vi "Motor Controller Config PID.vi"(0 "COM port":refnum<visa-resource-name>, 5 "RS-485 addr.":u8, 7 "Command":string(combo)="Q", 9 "PID params":T1={"N bits"=13, "dt (s)"=0.002, "Kp (/rpm)"=0.002, "Ti (s)"=0.01, "Td (s)"=0.0} {"N bits" min=8 max=16 step=1; "Td (s)" format="%#_6f"; "Ti (s)" format="%#_6f"; "Kp (/rpm)" format="%#_6f"; "dt (s)" format="%#_6f"}, 11 "Set as power-on default":bool, 12 "Close port after action":bool) -> (4 "COM port out":refnum<visa-resource-name>, 15 "Error out":errorcluster)   [LabVIEW 2020]
uses:
  ctls/CTRL_PID_params.ctl
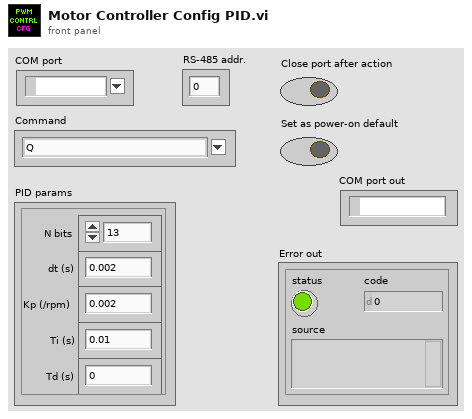
[diagram p1: front panel]
types:
  T1 = typedef "CTRL_PID_params.ctl" = cluster{"N bits":u8, "dt (s)":sgl, "Kp (/rpm)":sgl, "Ti (s)":sgl, "Td (s)":sgl}
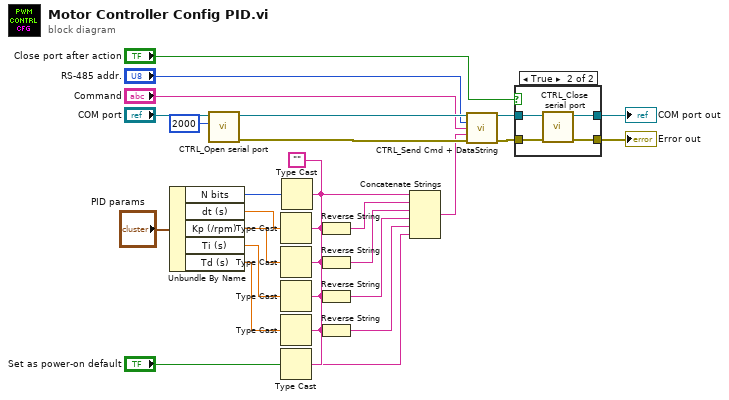
[diagram p0: block diagram]
diagram:
  w5 = ""
  n1 = Unbundle By Name("PID params") -> ("N bits"=w8:u8, "dt (s)"=w14:sgl, "Kp (/rpm)"=w13:sgl, "Ti (s)"=w12:sgl, "Td (s)"=w11:sgl)
  n2 = call "CTRL_Open serial port.vi"("timeout (ms)"=u32 2000, "VISA resource name"="COM port") -> ("Error out"=w27:errorcluster, "VISA resource name out"=w28:refnum<visa-resource-name>)  [unwired: 8 in]
  n3 = Type Cast(type=w5, x=w14) -> (*(type *) &x=w22:string)
  n4 = Type Cast(type=w5, x=w13) -> (*(type *) &x=w21:string)
  n5 = Type Cast(type=w5, x=w12) -> (*(type *) &x=w19:string)
  n6 = Type Cast(type=w5, x=w11) -> (*(type *) &x=w20:string)
  n7 = Type Cast(type=w5, x="Set as power-on default") -> (*(type *) &x=w4:string)
  n8 = Type Cast(type=w5, x=w8) -> (*(type *) &x=w7:string)
  n9 = Reverse String(1:w22) -> (0:w18:string)
  n10 = Reverse String(1:w21) -> (0:w17:string)
  n11 = Reverse String(1:w19) -> (0:w16:string)
  n12 = Reverse String(1:w20) -> (0:w15:string)
  n13 = Concatenate Strings(w7, w18, w17, w16, w15, w4) -> (w10:string)
  n14 = call "CTRL_Send Cmd + DataString.vi"("Port"=w28, "RS-485 addr."="RS-485 addr.", "Cmd"="Command", "DataString"=w10, "Error In"=w27) -> ("Port out"=w25:refnum<visa-resource-name>, "Error Out"=w24:errorcluster)  [unwired: 9 in]
  n15 = case shown="True" "Close port after action" {
    tunnel: [w32 w35] -> w26
    tunnel: w25 -> [w31 w33]
    tunnel: w24 -> [w32 w34]
    tunnel: [w31 w33] -> w1
    frame False {
    }
    frame True {
      n16 = call "CTRL_Close serial port.vi"("Error in"=w34, "VISA resource name"=w33) -> ("Error out"=w35:errorcluster)  [unwired: 9 in]
    }
  }
  "Error out" <- w26
  "COM port out" <- w1
